vi "Interface_RW.vi"(7 "Mode":enum16{"Write", "Read"}(ring), 8 "error in (no error)":errorcluster, 9 "In_IP Address":T1 caption="IN_Info_IP Address" {"Manual_IP"."IP4" format="%.03d"; "Manual_IP"."IP3" format="%.03d"; "Manual_IP"."IP2" format="%.03d"; "Manual_IP"."IP1" format="%.03d"; "Auto_IP"."IP3" format="%.03d"; "Auto_IP"."IP2" format="%.03d"; "Auto_IP"."IP1" format="%.03d"}, 10 "In_InterfaceCode":u32 caption="nInterfaceCode" format="%.0x") -> (0 "error out":errorcluster, 1 "Out_IP Address":T1 caption="Out_Info_IP Address" {"Manual_IP"."IP4" format="%.03d"; "Manual_IP"."IP3" format="%.03d"; "Manual_IP"."IP2" format="%.03d"; "Manual_IP"."IP1" format="%.03d"; "Auto_IP"."IP3" format="%.03d"; "Auto_IP"."IP2" format="%.03d"; "Auto_IP"."IP1" format="%.03d"}, 2 "Out_InterfaceCode":u32 caption="nInterfaceCode" format="%.0x")   [LabVIEW 2015]
uses:
  <vilib>/Utility/config.llb/Write Key (String).vi
  <vilib>/Utility/config.llb/Read Key (String).vi
  <vilib>/Utility/config.llb/NI_LVConfig.lvlib
panel:
  # "．"
  # "．"
  # "．"
  # "．"
  # "．"
  # "．"
  # "XXX"
  # "．"
  # "．"
  # "．"
  # "．"
  # "．"
  # "．"
  # "XXX"
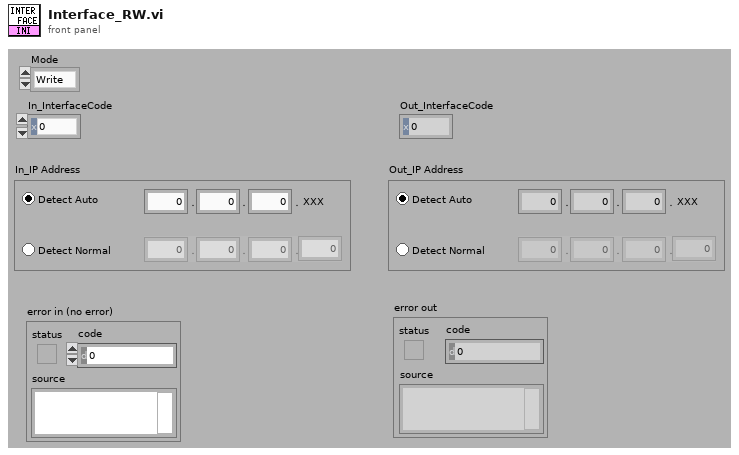
[diagram p1: front panel]
types:
  T1 = cluster{"Detect Select BOX":enum32{"Detect Auto", "Detect Normal"}, "Auto_IP":cluster{"IP1":u8, "IP2":u8, "IP3":u8}, "Manual_IP":cluster{"IP1":u8, "IP2":u8, "IP3":u8, "IP4":u8}}
  T2 = typedef "NI_LVConfig.lvlib/Config Data RefNum.ctl" = refnum<k1>
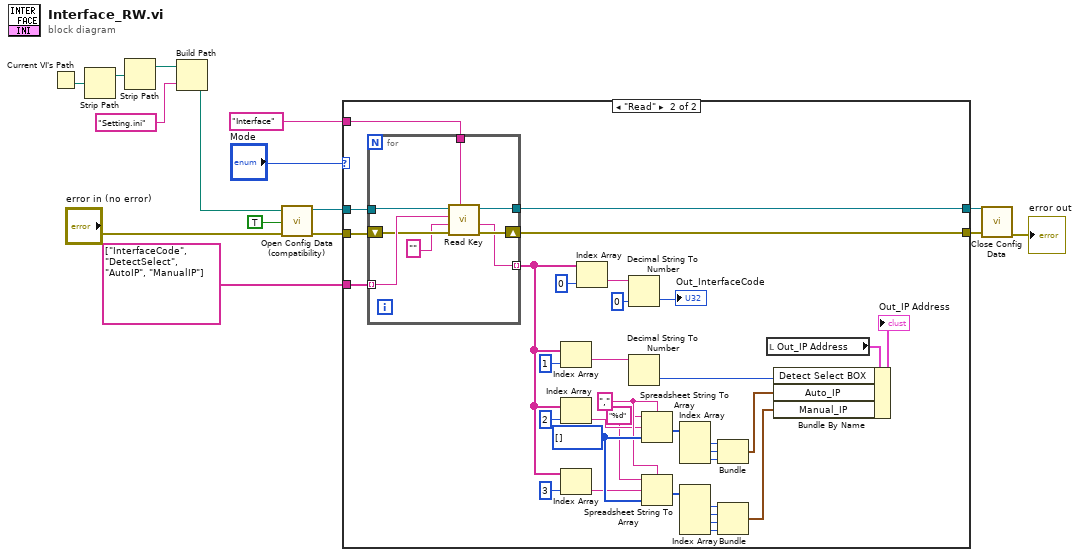
[diagram p0: block diagram]
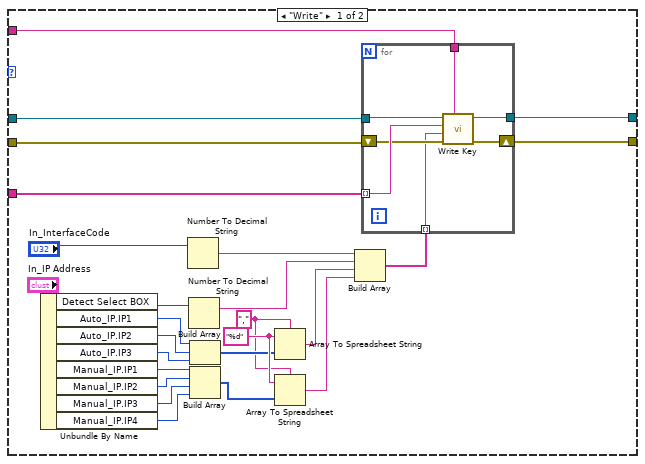
[diagram p2: hidden frame]
diagram:
  n1 = Current VI's Path() -> (path=w6:path)
  n2 = Strip Path(path=w6) -> (stripped path=w5:path)  [unwired: 1 out]
  n3 = Strip Path(path=w5) -> (stripped path=w4:path)  [unwired: 1 out]
  n4 = Build Path(base path=w4, name or relative path="Setting.ini" ("section")) -> (appended path=w2:path)
  n5 = call <vilib>:"Open Config Data (compatibility).vi"("error in (no error)"="error in (no error)", "create file if necessary (T)"=TRUE ("create file if necessary? (T)"), "configuration file path"=w2) -> ("error out"=w10:errorcluster, "refnum"=w14:T2)  [unwired: 6 in, 1 out]
  n6 = case shown="\"Read\"" "Mode" {
    tunnel: w14 -> [w40 w81]
    tunnel: string[] ["InterfaceCode", "DetectSelect", "AutoIP", "ManualIP"] -> [w39 w80]
    tunnel: [w38 w79] -> w12
    tunnel: w10 -> [w37 w78]
    tunnel: [w36 w77] -> w9
    tunnel: "Interface" ("section") -> [w35 w76]
    frame "Write" {
      w16 = ","
      w30 = "%d" ("形式文字列")
      n7 = Unbundle By Name("In_IP Address") -> ("Detect Select BOX"=w20:enum32{"Detect Auto", "Detect Normal"}, "Auto_IP.IP1"=w21:u8, "Auto_IP.IP2"=w22:u8, "Auto_IP.IP3"=w23:u8, "Manual_IP.IP1"=w24:u8, "Manual_IP.IP2"=w25:u8, "Manual_IP.IP3"=w26:u8, "Manual_IP.IP4"=w27:u8)
      n8 = Number To Decimal String(number="In_InterfaceCode") -> (decimal integer string=w31:string)  [unwired: 1 out]
      n9 = Number To Decimal String(number=w20) -> (decimal integer string=w33:string)  [unwired: 1 out]
      n10 = Build Array(w21, w22, w23) -> (w28:u8[])
      n11 = Build Array(w24, w25, w26, w27) -> (w29:u8[])
      n12 = Array To Spreadsheet String(delimiter (Tab)=w16, array=w28, 3:w30) -> (spreadsheet string=w32:string)
      n13 = Array To Spreadsheet String(delimiter (Tab)=w16, array=w29, 3:w30) -> (spreadsheet string=w34:string)
      n14 = Build Array(w31, w33, w32, w34) -> (w17:string[])
      n15 = for {
        tunnel: w40 -> [w47]
        tunnel: w35 -> [w46]
        tunnel: w39 -> [w45] mode=indexing
        tunnel: [w44] -> w38
        shift-right: [w42] -> w36
        shift-left: w37 -> [w43]
        tunnel: w17 -> [w41] mode=indexing
        n16 = call-poly <vilib>:"Write Key.vi"("section"=w46, "error in (no error)"=w43, "value"=w41, "key"=w45, "refnum"=w47) -> ("error out"=w42:errorcluster, "refnum out"=w44:T2)  [unwired: 1 in, 4 out]
      }
    }
    frame "Read" {
      w48 = "%d"
      w51 = ","
      w64 = u8[] [] ("配列タイプ（2次元Dbl）")
      n17 = for {
        tunnel: w81 -> [w89]
        tunnel: w76 -> [w88]
        tunnel: w80 -> [w87] mode=indexing
        tunnel: [w86] -> w79
        shift-right: [w84] -> w77
        shift-left: w78 -> [w85]
        tunnel: [w82] -> w68 mode=indexing
        n18 = call-poly <vilib>:"Read Key.vi"("section"=w88, "error in (no error)"=w85, "default value"="", "key"=w87, "refnum"=w89) -> ("error out"=w84:errorcluster, "value"=w82:string, "refnum out"=w86:T2)  [unwired: 1 in, 3 out]
      }
      n19 = Index Array(array=w68, index=1 ("指標")) -> (element=w66:string)
      n20 = Index Array(array=w68, index=2 ("指標")) -> (element=w50:string)
      n21 = Index Array(array=w68, index=3 ("指標")) -> (element=w49:string)
      n22 = Index Array(array=w68, index=0 ("指標")) -> (element=w71:string)
      n23 = Decimal String To Number(string=w71, default (0L)=u32 0 ("デフォルト (0 I32)")) -> (number=→"Out_InterfaceCode":u32)  [unwired: 2 out]
      n24 = Decimal String To Number(string=w66) -> (number=w65:i32)  [unwired: 3 out]
      n25 = Spreadsheet String To Array(delimiter (Tab)=w51, format string=w48, spreadsheet string=w50, array type (2D Dbl)=w64) -> (array=w63:u8[])
      n26 = Spreadsheet String To Array(delimiter (Tab)=w51, format string=w48, spreadsheet string=w49, array type (2D Dbl)=w64) -> (array=w56:u8[])
      n27 = Index Array(array=w63) -> (element #1=w62:u8, element #2=w61:u8, element #3=w60:u8)  [unwired: 3 in]
      n28 = Index Array(array=w56) -> (element #1=w57:u8, element #2=w58:u8, element #3=w59:u8, element #4=w55:u8)  [unwired: 4 in]
      n29 = Bundle(w62, w61, w60) -> (w54:cluster{u8, u8, u8})  [unwired: 1 out]
      n30 = Bundle(w57, w58, w59, w55) -> (w53:cluster{u8, u8, u8, u8})  [unwired: 1 out]
      n31 = local read "Out_IP Address"() -> (w67:T1)
      n32 = Bundle By Name(cluster=w67, "Detect Select BOX"=w65, "Auto_IP"=w54, "Manual_IP"=w53) -> (→"Out_IP Address":T1)
    }
  }
  n33 = call <vilib>:"Close Config Data.vi"("error in (no error)"=w9, "refnum"=w12) -> ("error out"=→"error out":errorcluster)  [unwired: 1 in, 8 out]
